vi "Untitled 1 (SubVI).vi"(10 "Array":dbl[](array[numeric]), 11 "dt":dbl) -> (3 "result":dbl)   [LabVIEW 2011]
uses:
  NI_AALBase.lvlib
  NI_AALPro.lvlib
panel:
  out "Filtered X 3":dbl[](graph)
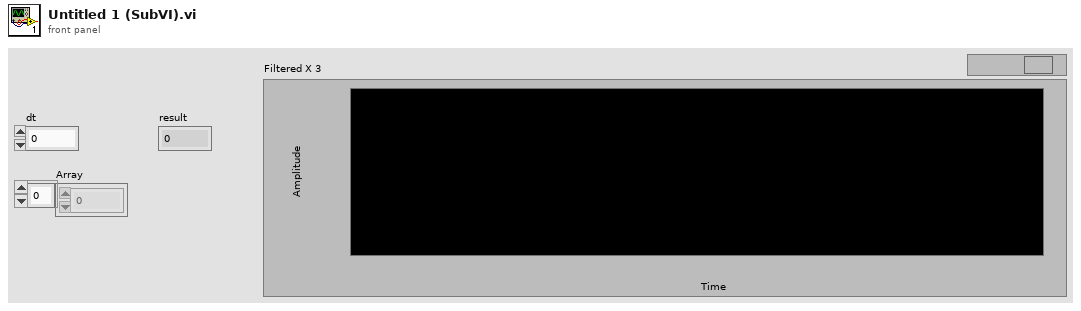
[diagram p1: front panel]
types:
  T1 = enum32{"Trapezoidal Rule", "Simpson's Rule", "Simpson's 3/8 Rule", "Bode Rule"}
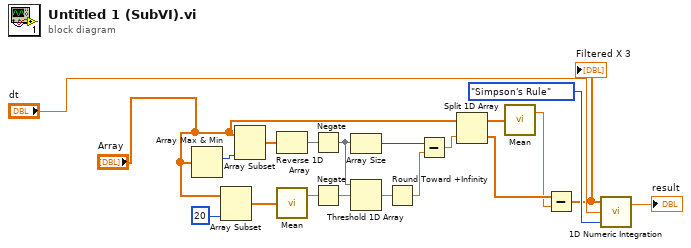
[diagram p0: block diagram]
diagram:
  n1 = Array Max & Min(array="Array") -> (max index (indices)=w6:i32)  [unwired: 3 out]
  n2 = Array Subset(array="Array", length=20) -> (w4:dbl[])  [unwired: 1 in]
  n3 = Array Subset(array="Array", length=w6) -> (w5:dbl[])  [unwired: 1 in]
  n4 = Reverse 1D Array(array=w5) -> (reversed array=w7:dbl[])
  n5 = call "Mean.vi"("X"=w4) -> ("mean"=w9:dbl)  [unwired: 1 out]
  n6 = Negate(x=w7) -> (-x=w8:dbl[])
  n7 = Negate(x=w9) -> (-x=w10:dbl)
  n8 = Array Size(array=w8) -> (size(s)=w11:i32)
  n9 = Threshold 1D Array(2:w10, 3:w8) -> (0:w14:dbl)  [unwired: 1 in]
  n10 = Round Toward +Infinity(x=w14) -> (ceil(x): smallest int >= x=w15:dbl)
  n11 = Subtract(x=w11, y=w15) -> (x-y=w16:dbl)
  n12 = Split 1D Array(array="Array", index=w16) -> (first subarray=w12:dbl[], second subarray=w19:dbl[])
  n13 = call "Mean.vi"("X"=w12) -> ("mean"=w13:dbl)  [unwired: 1 out]
  n14 = Subtract(x=w19, y=w13) -> (x-y=w2:dbl[])
  "Filtered X 3" <- w2
  n15 = call "1D Numeric Integration.vi"("integration method"=T1."Simpson's Rule", "dt"="dt", "Input Array"=w2) -> ("result"=→"result":dbl)  [unwired: 1 out]
